vi "Get All Channel Refs.vi"(8 "error in (no error)":errorcluster, 10 "framework configuration in":T1, 11 "VeriStand Data Sharing Framework in":refnum<class "VeriStand Data Sharing Framework.lvclass">=refnum) -> (0 "error out":errorcluster, 1 "contiguous?":bool, 2 "all channel offsets":u64[](array[numeric]) format="%.0x", 3 "VeriStand Data Sharing Framework out":refnum<class "VeriStand Data Sharing Framework.lvclass">)   [LabVIEW 2017, in "Data Sharing Framework Engine.lvlib" / "VeriStand Data Sharing Framework.lvclass"]
uses:
  VeriStand Data Sharing Framework.lvclass
  DSF Core.lvlibp/Typedefs/DSF Engine Framework Configuration.ctl
  DSF Core.lvlibp/Typedefs/DSF Engine Plugin Configuration.ctl
  DSF Core.lvlibp/Typedefs/DSF Timing Info.ctl
  DSF Core.lvlibp/Typedefs/DSF Engine Plugin Thread Configuration.ctl
  DSF Core.lvlibp/Typedefs/DSF Settings Info.ctl
  DSF Core.lvlibp/Typedefs/DSF Engine Transfer Group Configuration.ctl
  DSF Core.lvlibp/Typedefs/DSF Direction.ctl
  DSF Core.lvlibp/Typedefs/DSF Engine Transfer Configuration.ctl
  DSF Core.lvlibp/Typedefs/DSF Byte Order.ctl
  DSF Core.lvlibp/Typedefs/DSF Engine Channel Configuration.ctl
  DSF Core.lvlibp/Typedefs/DSF Data Type.ctl
  DSF Core.lvlibp/Typedefs/DSF Timeout Behavior.ctl
  VeriStand Data Sharing Framework.lvclass/VeriStand Data Sharing Framework.ctl
  <vilib>/NI Veristand/Custom Device API/Data Access Type.ctl
  DSF Core.lvlibp/Classes/Configuration/Channel Count (Transfer).vi
  <vilib>/NI Veristand/Custom Device API/Custom Device API.lvlib
  DSF Core.lvlibp
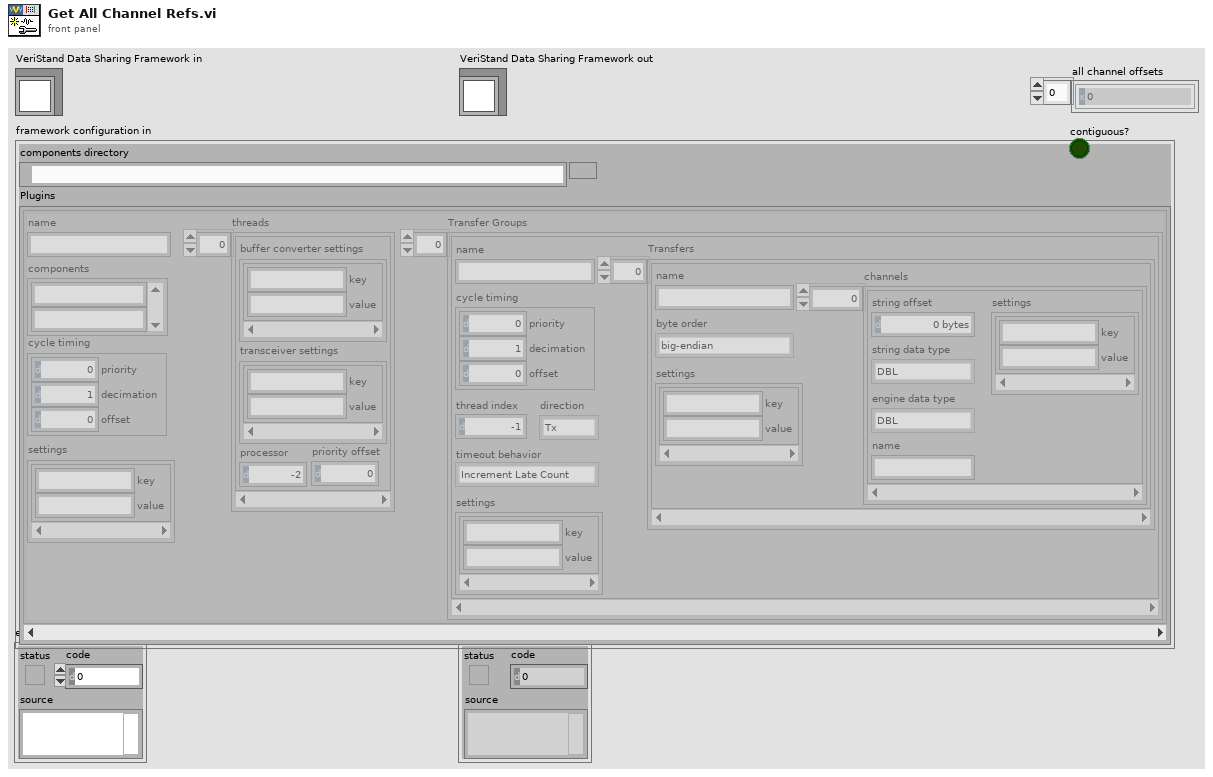
[diagram p1: front panel]
types:
  T1 = typedef "DSF Core.lvlibp/DSF Engine Framework Configuration.ctl" = cluster{"components directory":path, "Plugins":T2[]}
  T2 = typedef "DSF Core.lvlibp/DSF Engine Plugin Configuration.ctl" = cluster{"name":string, "components":string[], "cycle timing":T3, "threads":T4[], "Transfer Groups":T6[], "settings":T5}
  T3 = typedef "DSF Core.lvlibp/DSF Timing Info.ctl" = cluster{"priority":u64, "decimation":u64, "offset":u64}
  T4 = typedef "DSF Core.lvlibp/DSF Engine Plugin Thread Configuration.ctl" = cluster{"buffer converter settings":T5, "transceiver settings":T5, "processor":i32, "priority offset":i16}
  T5 = typedef "DSF Core.lvlibp/DSF Settings Info.ctl" = cluster{"key":string, "value":string}[]
  T6 = typedef "DSF Core.lvlibp/DSF Engine Transfer Group Configuration.ctl" = cluster{"name":string, "direction":T7, "cycle timing":T3, "thread index":i32, "settings":T5, "Transfers":T8[], "timeout behavior":T12}
  T7 = typedef "DSF Core.lvlibp/DSF Direction.ctl" = enum8{"Tx", "Rx"}
  T8 = typedef "DSF Core.lvlibp/DSF Engine Transfer Configuration.ctl" = cluster{"name":string, "byte order":T9, "settings":T5, "channels":T10[]}
  T9 = typedef "DSF Core.lvlibp/DSF Byte Order.ctl" = enum8{"big-endian", "little-endian"}
  T10 = typedef "DSF Core.lvlibp/DSF Engine Channel Configuration.ctl" = cluster{"string offset":u64, "string data type":T11, "engine data type":T11, "name":string, "settings":T5}
  T11 = typedef "DSF Core.lvlibp/DSF Data Type.ctl" = enum8{"Bool", "SGL", "DBL", "I8", "I16", "I32", "I64", "U8", "U16", "U32", "U64"}
  T12 = typedef "DSF Core.lvlibp/DSF Timeout Behavior.ctl" = enum8{"Increment Late Count", "Throw Error"}
  T13 = typedef "Custom Device API.lvlib/Custom Device Item Ref.ctl" = u64
  T14 = typedef "Custom Device API.lvlib/Data Access Type.ctl" = enum16{"Read", "Write"}
  T15 = typedef "Custom Device API.lvlib/Data Reference.ctl" = i32
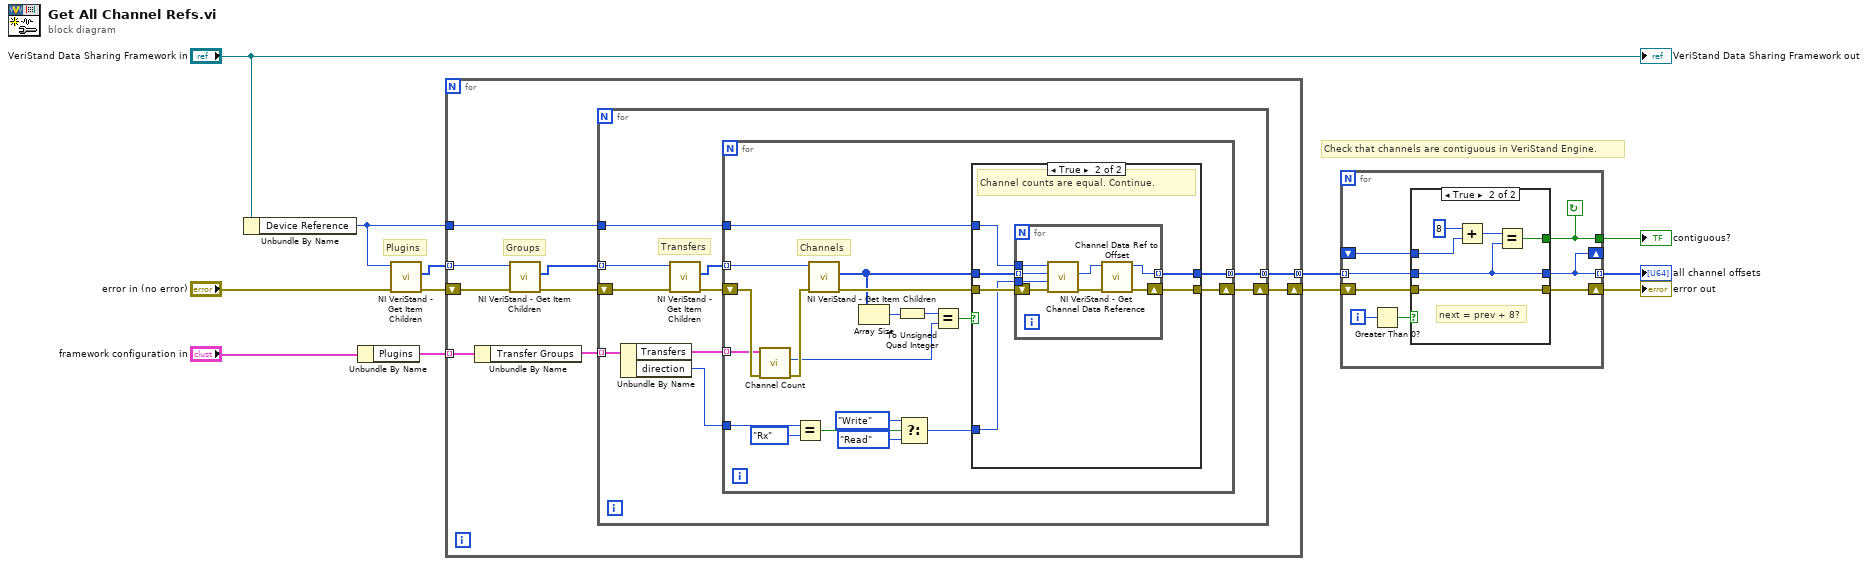
[diagram p0: block diagram]
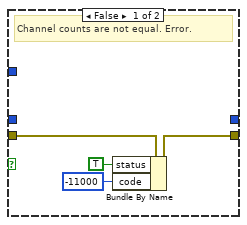
[diagram p2: hidden frame]
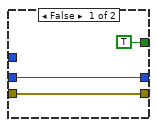
[diagram p3: hidden frame]
diagram:
  # "Check that channels are contiguous in VeriStand Engine."
  # "Plugins"
  n1 = Unbundle By Name("VeriStand Data Sharing Framework in") -> ("Device Reference"=w8:T13)
  n2 = Unbundle By Name("framework configuration in") -> ("Plugins"=w9:T2[])
  n3 = call <vilib>:"NI VeriStand - Get Item Children.vi"("error in (no error)"="error in (no error)", "Item Ref in"=w8) -> ("error out"=w7:errorcluster, "Child Refs"=w10:T13[])  [unwired: 6 in, 2 out]
  n4 = for {
    tunnel: w10 -> [w20] mode=indexing
    tunnel: w9 -> [w21] mode=indexing
    tunnel: w8 -> [w19]
    shift-right: [w17] -> w5
    shift-left: w7 -> [w18]
    tunnel: [w16] -> w4 mode=concatenating
    # "Groups"
    n5 = Unbundle By Name(w21) -> ("Transfer Groups"=w15:T6[])
    n6 = call <vilib>:"NI VeriStand - Get Item Children.vi"("error in (no error)"=w18, "Item Ref in"=w20) -> ("error out"=w13:errorcluster, "Child Refs"=w14:T13[])  [unwired: 6 in, 2 out]
    n7 = for {
      tunnel: w15 -> [w30] mode=indexing
      tunnel: w14 -> [w31] mode=indexing
      tunnel: w19 -> [w29]
      shift-right: [w27] -> w17
      shift-left: w13 -> [w28]
      tunnel: [w26] -> w16 mode=concatenating
      # "Transfers"
      n8 = Unbundle By Name(w30) -> ("Transfers"=w25:T8[], "direction"=w22:T7)
      n9 = call <vilib>:"NI VeriStand - Get Item Children.vi"("error in (no error)"=w28, "Item Ref in"=w31) -> ("error out"=w23:errorcluster, "Child Refs"=w24:T13[])  [unwired: 6 in, 2 out]
      n10 = for {
        tunnel: w25 -> [w34] mode=indexing
        tunnel: w24 -> [w50] mode=indexing
        tunnel: w22 -> [w48]
        tunnel: w29 -> [w41]
        shift-right: [w33] -> w27
        shift-left: w23 -> [w37]
        tunnel: [w32] -> w26 mode=concatenating
        # "Channels"
        n11 = call-poly "Channel Count.vi"("error in (no error)"=w37, "Transfer Configuration in"=w34) -> ("error out"=w36:errorcluster, "total channel count"=w35:u64)  [unwired: 7 in, 1 out]
        n12 = Equal?(x=w48, y=DSF_Direction."Rx") -> (x = y?=w46:bool)
        n13 = call <vilib>:"NI VeriStand - Get Item Children.vi"("error in (no error)"=w36, "Item Ref in"=w50) -> ("error out"=w39:errorcluster, "Child Refs"=w38:T13[])  [unwired: 6 in, 2 out]
        n14 = Array Size(array=w38) -> (size(s)=w49:i32)
        n15 = To Unsigned Quad Integer(1:w49) -> (0:w42:u64)
        n16 = Select(t=Data_Access_Type."Write" ("Access"), s=w46, f=Data_Access_Type."Read") -> (s? t:f=w40:T14)
        n17 = Equal?(x=w42, y=w35) -> (x = y?=w43:bool)
        n18 = case shown="True" w43 {
          tunnel: w38 -> [_ w57]
          tunnel: w41 -> [_ w59]
          tunnel: w40 -> [_ w58]
          tunnel: w39 -> [w54 w60]
          tunnel: [w53 w55] -> w33
          tunnel: [_ w56] -> w32
          frame False {
            # "Channel counts are not equal. Error."
            n19 = Bundle By Name(cluster=w54, "status"=TRUE, "code"=-11000) -> (w53:errorcluster)
          }
          frame True {
            # "Channel counts are equal. Continue."
            n20 = for {
              tunnel: w59 -> [w67]
              tunnel: w58 -> [w66]
              tunnel: w57 -> [w65] mode=indexing
              tunnel: [w61] -> w56 mode=indexing
              shift-right: [w62] -> w55
              shift-left: w60 -> [w68]
              n21 = call <vilib>:"NI VeriStand - Get Channel Data Reference.vi"("error in (no error)"=w68, "Access"=w66, "Channel Ref in"=w65, "Device Ref in"=w67) -> ("error out"=w64:errorcluster, "Channel Data Reference"=w63:T15)  [unwired: 5 in, 1 out]
              n22 = call "Channel Data Ref to Offset.vi"("error in (no error)"=w64, "Channel Data Reference"=w63) -> ("error out"=w62:errorcluster, "channel offset"=w61:u64)  [unwired: 8 in]
            }
          }
        }
      }
    }
  }
  n23 = for {
    tunnel: w4 -> [w74] mode=indexing
    shift-right: [w71] -> w3
    shift-left: w5 -> [w73]
    shift-right: [w69] -> _
    shift-left: _ -> [w72]
    tunnel: [w70] -> w2
    tunnel: [w69] -> w1 mode=indexing
    i -> [w76]
    stop <- w70 continue-if-true
    n24 = Greater Than 0?(x=w76) -> (x > 0?=w75:bool)
    n25 = case shown="True" w75 {
      tunnel: w74 -> [w78 w81]
      tunnel: w73 -> [w79 w80]
      tunnel: w72 -> [_ w85]
      tunnel: [w79 w80] -> w71
      tunnel: [TRUE w82] -> w70
      tunnel: [w78 w81] -> w69
      frame False {
      }
      frame True {
        # "next = prev + 8?"
        n26 = Add(x=u64 8 ("y"), y=w85) -> (x+y=w83:u64)
        n27 = Equal?(x=w83, y=w81) -> (x = y?=w82:bool)
      }
    }
  }
  "error out" <- w3
  "all channel offsets" <- w1
  "contiguous?" <- w2
  "VeriStand Data Sharing Framework out" <- "VeriStand Data Sharing Framework in"
